vi "Add Caption and Table V2.vi"(0 "PDF Report IN":refnum<class "PDF Report Class.lvclass">, 2 "Caption?":bool, 5 "PdfpTable Title Refnum":refnum<k24>, 7 "PdfPTable":refnum<k24>, 11 "error in (no error)":errorcluster) -> (4 "PDF Report OUT":refnum<class "PDF Report Class.lvclass">, 15 "error out":errorcluster)   [LabVIEW 2019]
doc: "Version 2.0\nDeveloped by Jean-Marc Simard\nCopyright © 2012, Exaprom Inc.\nAll rights reserved.\nLicense: BSD\n\nWith iTextSharp 4.1.6 (http://itextsharp.sourceforge.net)\nunder Mozilla Public License Version 1.1\n(http://www.mozilla.org/MPL/MPL-1.1.html)"
uses:
  <userlib>/Exaprom PDF/LV Class/PDF Report Class/PDF Report Class.lvclass
  C:/Program Files/National Instruments/LabVIEW 2019/user.lib/Exaprom PDF/DLL/itextsharp.dll
  DLL/itextsharp.dll
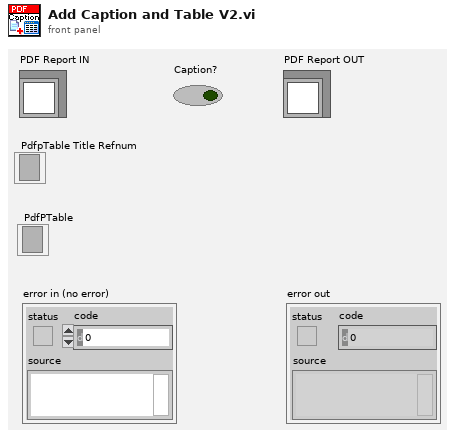
[diagram p1: front panel]
types:
  T1 = typedef "Captions.ctl" = cluster{"Figure":T2, "Table":T2, "Font":T3}
  T2 = typedef "Image or Table Caption.ctl" = cluster{"Caption":string, "Separator":string, "Position":enum16{"Above", "Below"}}
  T3 = typedef "Font complete cluster.ctl" = cluster{"Name":string, "Size":T4, "Color":T5, "Style":cluster{"Bold":bool, "Italic":bool, "Underline":bool, "Strikeout":bool}, "Type":T6}
  T4 = typedef "Font size.ctl" = sgl
  T5 = typedef "Font color.ctl" = u32
  T6 = typedef "Type and encoding.ctl" = cluster{"Type&direction":T7, "Embedded":bool, "Encoding":string}
  T7 = typedef "Type and run direction.ctl" = enum16{"Select", "ASCII", "UTF-16", "UTF-16 (default)", "UTF-16 (LTR)", "UTF-16 (RTL)"}
  T8 = cluster{"Captions":T1, "Image counter":u16, "Table counter":u16}
  T9 = cluster{"HorizontalAlignment":i32, "SpacingBefore":sgl, "SpacingAfter":sgl}
  T10 = cluster{"HorizontalAlignment":i32, "SpacingAfter":sgl, "SpacingAfter":sgl}
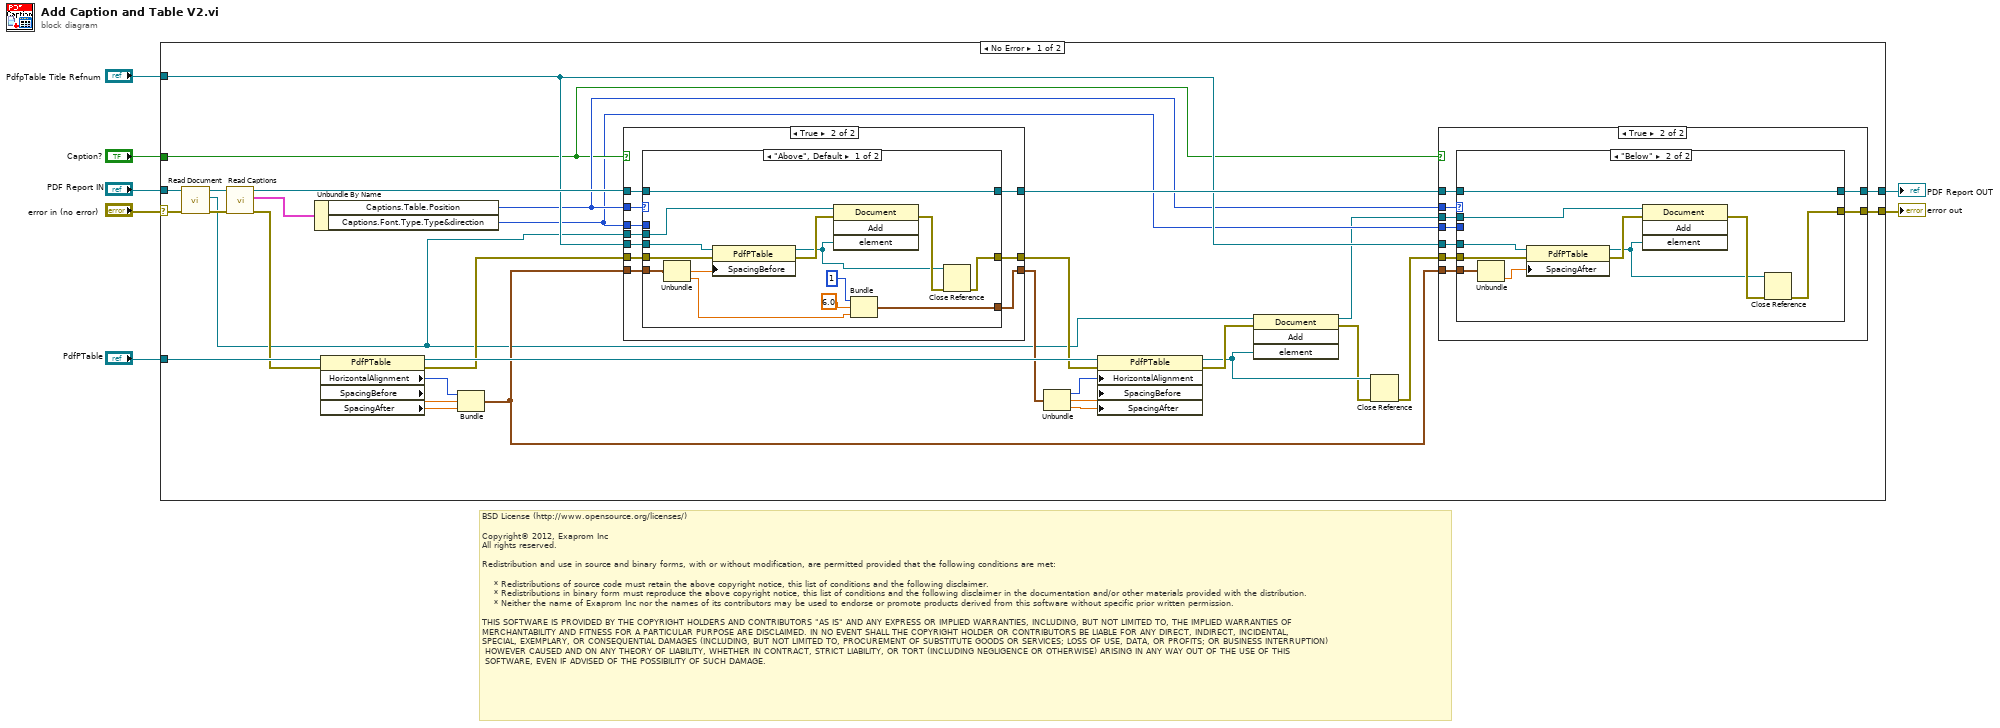
[diagram p0: block diagram]
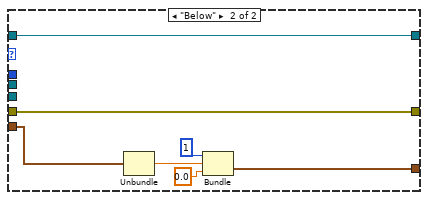
[diagram p5: hidden frame]
diagram:
  # "BSD License (http://www.opensource.org/licenses/)\n\nCopyright© 2012, Exaprom Inc\nAll rights reserved.\n\nRedistribution and use in source and binary forms, with or without modification, are permitted provided that the following conditions are met:\n\n    * Redistributions of source code must retain the above copyright notice, this list of conditions and the following disclaimer.\n    * Redistributions in binary form must reproduce the above copyright notice, this list of conditions and the following disclaimer in the documentation and/or other materials provided with the distribution.\n    * Neither the name of Exaprom Inc nor the names of its contributors may be used to endorse or promote products derived from this software without specific prior written permission.\n\nTHIS SOFTWARE IS PROVIDED BY THE COPYRIGHT HOLDERS AND CONTRIBUTORS \"AS IS\" AND ANY EXPRESS OR IMPLIED WARRANTIES, INCLUDING, BUT NOT LIMITED TO, THE IMPLIED WARRANTIES OF \nMERCHANTABILITY AND FITNESS FOR A PARTICULAR PURPOSE ARE DISCLAIMED. IN NO EVENT SHALL THE COPYRIGHT HOLDER OR CONTRIBUTORS BE LIABLE FOR ANY DIRECT, INDIRECT, INCIDENTAL,\nSPECIAL, EXEMPLARY, OR CONSEQUENTIAL DAMAGES (INCLUDING, BUT NOT LIMITED TO, PROCUREMENT OF SUBSTITUTE GOODS OR SERVICES; LOSS OF USE, DATA, OR PROFITS; OR BUSINESS INTERRUPTION)\n HOWEVER CAUSED AND ON ANY THEORY OF LIABILITY, WHETHER IN CONTRACT, STRICT LIABILITY, OR TORT (INCLUDING NEGLIGENCE OR OTHERWISE) ARISING IN ANY WAY OUT OF THE USE OF THIS\n SOFTWARE, EVEN IF ADVISED OF THE POSSIBILITY OF SUCH DAMAGE."
  n1 = case shown="No Error" "error in (no error)" {
    selector: "error in (no error)" -> [w24 w98]
    tunnel: "PDF Report IN" -> [w28 w97]
    tunnel: [w12 w97] -> w6
    tunnel: [w11 w98] -> w5
    tunnel: "PdfPTable" -> [w29 _]
    tunnel: "Caption?" -> [w13 _]
    tunnel: "PdfpTable Title Refnum" -> [w15 _]
    frame No Error {
      n2 = call-dynamic "Read Document.vi"("error in (no error)"=w24, "PDF Report Class in"=w28) -> ("error out"=w26:errorcluster, "Document"=w9:refnum<k24>, "PDF Report Class out"=w25:refnum<class "PDF Report Class.lvclass">)  [unwired: 7 in]
      n3 = call-dynamic "Read Captions.vi"("error in (no error)"=w26, "PDF Report Class in"=w25) -> ("error out"=w23:errorcluster, "Captions and counters"=w27:T8, "PDF Report Class out"=w21:refnum<class "PDF Report Class.lvclass">)  [unwired: 7 in]
      n4 = Unbundle By Name(w27) -> ("Captions.Table.Position"=w14:enum16{"Above", "Below"}, "Captions.Font.Type.Type&direction"=w10:T7)
      n5 = property class="PdfPTable"(reference=w29, error in=w23) -> (reference out=w39:refnum<k24>, error out=w22:errorcluster, "HorizontalAlignment"=w36:i32, "SpacingBefore"=w37:sgl, "SpacingAfter"=w38:sgl)
      n6 = Bundle("HorizontalAlignment"=w36, "SpacingBefore"=w37, "SpacingAfter"=w38) -> (w16:T9)  [unwired: 1 out]
      n7 = case shown="True" w13 {
        tunnel: w22 -> [w65 w75]
        tunnel: [w65 w74] -> w19
        tunnel: w14 -> [_ w73]
        tunnel: w15 -> [_ w72]
        tunnel: w21 -> [w64 w71]
        tunnel: [w64 w70] -> w18
        tunnel: w10 -> [_ w69]
        tunnel: w16 -> [w63 w68]
        tunnel: [w63 w67] -> w20
        tunnel: w9 -> [_ w66]
        frame False {
        }
        frame True {
          n8 = case shown="\"Above\", Default" w73 {
            tunnel: w72 -> [w86 _]
            tunnel: w75 -> [w87 w96]
            tunnel: [w78 w96] -> w74
            tunnel: w71 -> [w81 w95]
            tunnel: [w81 w95] -> w70
            tunnel: w69 -> [_ _]
            tunnel: w68 -> [w88 w90]
            tunnel: [w82 w91] -> w67
            tunnel: w66 -> [w79 _]
            frame "Above", Default {
              n9 = Unbundle(w88) -> ("SpacingBefore"=w89:sgl, "SpacingAfter"=w83:sgl)  [unwired: 1 out]
              n10 = property class="PdfPTable"(reference=w86, error in=w87, "SpacingBefore"=w89) -> (reference out=w76:refnum<k24>, error out=w80:errorcluster)
              n11 = invoke class="Document" method="Add"(reference=w79, error in=w80, "element"=w76) -> (error out=w77:errorcluster)  [unwired: 1 in, 3 out]
              n12 = Bundle("HorizontalAlignment"=1, "SpacingAfter"=sgl 6.0, "SpacingAfter"=w83) -> (w82:T10)  [unwired: 1 out]
              n13 = Close Reference(reference=w76, error in (no error)=w77) -> (error out=w78:errorcluster)
            }
            frame "Below" {
              n14 = Unbundle(w90) -> ("SpacingBefore"=w93:sgl)  [unwired: 2 out]
              n15 = Bundle("HorizontalAlignment"=1, "SpacingBefore"=w93, "SpacingAfter"=sgl 0.0) -> (w91:T9)  [unwired: 1 out]
            }
          }
        }
      }
      n16 = Unbundle(w20) -> ("HorizontalAlignment"=w33:i32, "SpacingBefore"=w34:sgl, "SpacingAfter"=w35:sgl)
      n17 = property class="PdfPTable"(reference=w39, error in=w19, "HorizontalAlignment"=w33, "SpacingBefore"=w34, "SpacingAfter"=w35) -> (reference out=w31:refnum<k24>, error out=w32:errorcluster)
      n18 = invoke class="Document" method="Add"(reference=w9, error in=w32, "element"=w31) -> (reference out=w8:refnum<k24>, error out=w30:errorcluster)  [unwired: 1 in, 2 out]
      n19 = Close Reference(reference=w31, error in (no error)=w30) -> (error out=w17:errorcluster)
      n20 = case shown="True" w13 {
        tunnel: w17 -> [w41 w50]
        tunnel: [w41 w49] -> w11
        tunnel: w14 -> [_ w48]
        tunnel: w15 -> [_ w47]
        tunnel: w18 -> [w40 w46]
        tunnel: [w40 w45] -> w12
        tunnel: w10 -> [_ w44]
        tunnel: w16 -> [_ w43]
        tunnel: w8 -> [_ w42]
        frame False {
        }
        frame True {
          n21 = case shown="\"Below\"" w48 {
            tunnel: w47 -> [_ w60]
            tunnel: w50 -> [w52 w61]
            tunnel: [w52 w54] -> w49
            tunnel: w46 -> [w51 w57]
            tunnel: [w51 w57] -> w45
            tunnel: w44 -> [_ _]
            tunnel: w43 -> [_ w62]
            tunnel: w42 -> [_ w56]
            frame "Above", Default {
            }
            frame "Below" {
              n22 = Unbundle(w62) -> ("SpacingAfter"=w59:sgl)  [unwired: 2 out]
              n23 = property class="PdfPTable"(reference=w60, error in=w61, "SpacingAfter"=w59) -> (reference out=w53:refnum<k24>, error out=w58:errorcluster)
              n24 = invoke class="Document" method="Add"(reference=w56, error in=w58, "element"=w53) -> (error out=w55:errorcluster)  [unwired: 1 in, 3 out]
              n25 = Close Reference(reference=w53, error in (no error)=w55) -> (error out=w54:errorcluster)
            }
          }
        }
      }
    }
    frame Error {
    }
  }
  "PDF Report OUT" <- w6
  "error out" <- w5
